vi "getSeries_from_node.vi"(8 "Error IN":errorcluster, 10 "Selected item":string, 11 "HEKAdat.lvclass IN":refnum<class "HEKAdat.lvclass">) -> (0 "Error OUT":errorcluster, 1 "File Parameters OUT":T1, 2 "Traces":sgl[][](array[numeric]), 3 "HEKAdat.lvclass OUT":refnum<class "HEKAdat.lvclass">)   [LabVIEW 2017, in "HEKAdat.lvclass"]
uses:
  HEKAdat.lvclass
  File Parameters.ctl
  HEKAdat.lvclass/HEKAdat.ctl
panel:
  in  "File Parameters":T1
  out "Dim_trace":i32[](array[numeric])
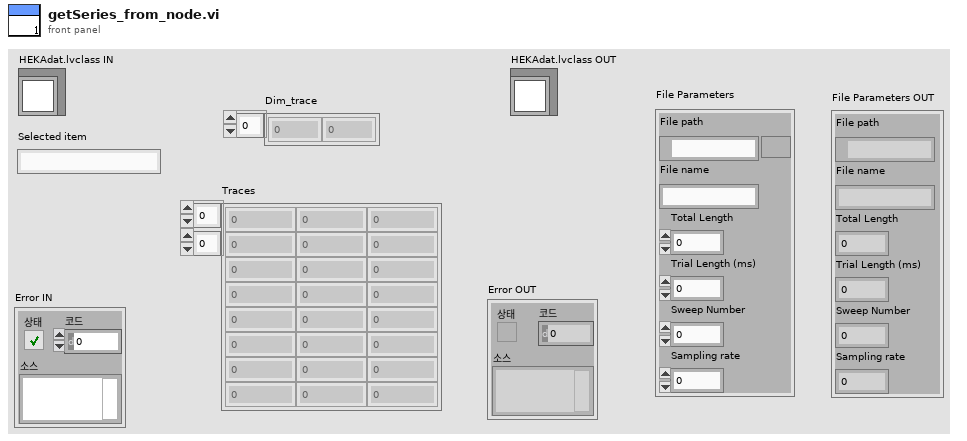
[diagram p1: front panel]
types:
  T1 = typedef "File Parameters.ctl" = cluster{"File path":path, "File name":string, "Total Length":i32, "Trial Length (ms)":dbl, "Sweep Number":dbl, "Sampling rate":dbl}
  T2 = cluster{"Label (Group)":string, "dataptr (Group)":u32, "nchildren (Group)":u32, "Series (1D)":cluster{"Label (Series)":string, "dataptr (Series)":u32, "nchildren (Series)":u32, "Sweep (1D)":cluster{"Label (Sweep)":string, "dataptr (Sweep)":u32, "nchildren (Sweep)":u32, "Trace (1D)":cluster{"dataptr (trace)":u32, "Label (Trace)":string, "Unit":string, "Unit_":dbl, "Xinterval":dbl, "nDatapoints":u32, "offset":u32, "Datascaler":dbl, "Trace":dbl[]}[]}[]}[]}[]
  T3 = cluster{"Label (Group)":string, "dataptr (Group)":u32, "nchildren (Group)":u32, "Series (1D)":cluster{"Label (Series)":string, "dataptr (Series)":u32, "nchildren (Series)":u32, "Sweep (1D)":cluster{"Label (Sweep)":string, "dataptr (Sweep)":u32, "nchildren (Sweep)":u32, "Trace (1D)":cluster{"dataptr (trace)":u32, "Label (Trace)":string, "Unit":string, "Unit_":dbl, "Xinterval":dbl, "nDatapoints":u32, "offset":u32, "Datascaler":dbl, "Trace":dbl[]}[]}[]}[]}
  T4 = cluster{"Label (Series)":string, "dataptr (Series)":u32, "nchildren (Series)":u32, "Sweep (1D)":cluster{"Label (Sweep)":string, "dataptr (Sweep)":u32, "nchildren (Sweep)":u32, "Trace (1D)":cluster{"dataptr (trace)":u32, "Label (Trace)":string, "Unit":string, "Unit_":dbl, "Xinterval":dbl, "nDatapoints":u32, "offset":u32, "Datascaler":dbl, "Trace":dbl[]}[]}[]}[]
  T5 = cluster{"Label (Series)":string, "dataptr (Series)":u32, "nchildren (Series)":u32, "Sweep (1D)":cluster{"Label (Sweep)":string, "dataptr (Sweep)":u32, "nchildren (Sweep)":u32, "Trace (1D)":cluster{"dataptr (trace)":u32, "Label (Trace)":string, "Unit":string, "Unit_":dbl, "Xinterval":dbl, "nDatapoints":u32, "offset":u32, "Datascaler":dbl, "Trace":dbl[]}[]}[]}
  T6 = cluster{"Label (Sweep)":string, "dataptr (Sweep)":u32, "nchildren (Sweep)":u32, "Trace (1D)":cluster{"dataptr (trace)":u32, "Label (Trace)":string, "Unit":string, "Unit_":dbl, "Xinterval":dbl, "nDatapoints":u32, "offset":u32, "Datascaler":dbl, "Trace":dbl[]}[]}[]
  T7 = cluster{"dataptr (trace)":u32, "Label (Trace)":string, "Unit":string, "Unit_":dbl, "Xinterval":dbl, "nDatapoints":u32, "offset":u32, "Datascaler":dbl, "Trace":dbl[]}[]
  T8 = cluster{"dataptr (trace)":u32, "Label (Trace)":string, "Unit":string, "Unit_":dbl, "Xinterval":dbl, "nDatapoints":u32, "offset":u32, "Datascaler":dbl, "Trace":i16[]}
  T9 = cluster{"Label (Sweep)":string, "dataptr (Sweep)":u32, "nchildren (Sweep)":u32, "Trace (1D)":cluster{"dataptr (trace)":u32, "Label (Trace)":string, "Unit":string, "Unit_":dbl, "Xinterval":dbl, "nDatapoints":u32, "offset":u32, "Datascaler":dbl, "Trace":dbl[]}[]}
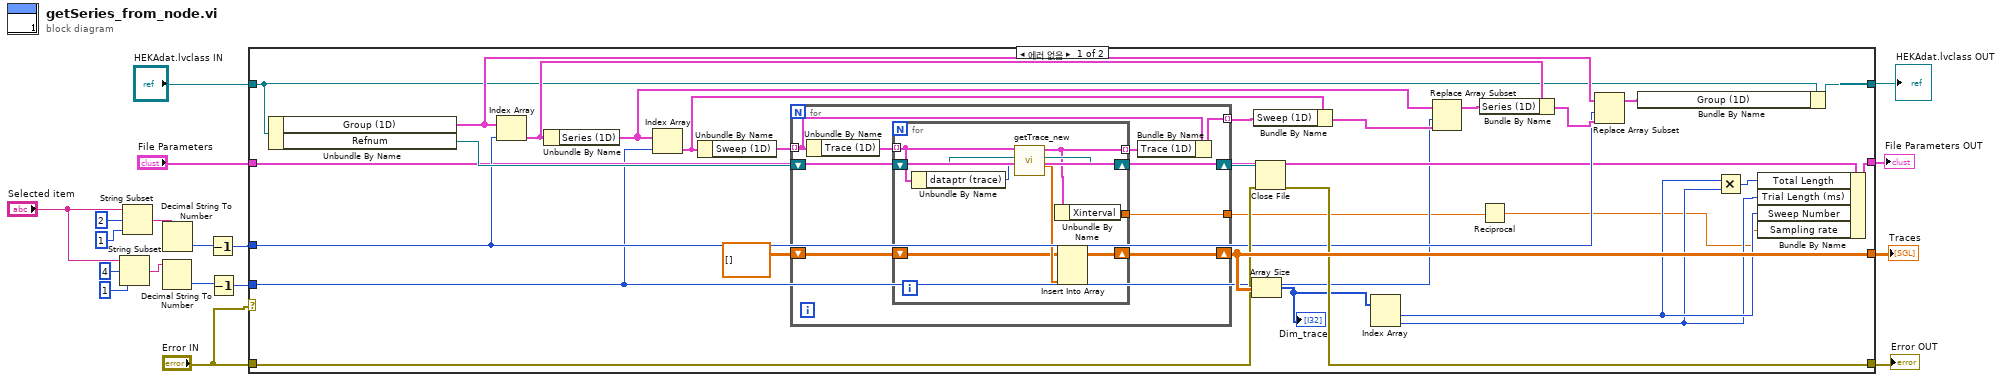
[diagram p0: block diagram]
diagram:
  n1 = String Subset(string="Selected item", offset (0)=4 ("오프셋(0)"), length (rest)=1 ("길이(나머지)")) -> (substring=w7:string)
  n2 = String Subset(string="Selected item", offset (0)=2 ("오프셋(0)"), length (rest)=1 ("길이(나머지)")) -> (substring=w8:string)
  n3 = Decimal String To Number(string=w7) -> (number=w3:i32)  [unwired: 2 in, 1 out]
  n4 = Decimal String To Number(string=w8) -> (number=w6:i32)  [unwired: 2 in, 1 out]
  n5 = Decrement(x=w6) -> (x-1=w5:i32)
  n6 = Decrement(x=w3) -> (x-1=w4:i32)
  n7 = case shown="에러 없음" "Error IN" {
    tunnel: "Error IN" -> [w41 w66]
    tunnel: [w40 w66] -> w17
    tunnel: "HEKAdat.lvclass IN" -> [w29 w65]
    tunnel: [w28 w65] -> w15
    tunnel: w5 -> [w31 _]
    tunnel: w4 -> [w25 _]
    tunnel: [w44 _] -> w14
    tunnel: "File Parameters" -> [w27 _]
    tunnel: [w26 _] -> w1
    frame No Error {
      n8 = Unbundle By Name(w29) -> ("Group (1D)"=w33:T2, "Refnum"=w43:refnum<file>)
      n9 = Index Array(array=w33, index=w31) -> (element=w35:T3)
      n10 = Unbundle By Name(w35) -> ("Series (1D)"=w37:T4)
      n11 = Index Array(array=w37, index=w25) -> (element=w39:T5)
      n12 = Unbundle By Name(w39) -> ("Sweep (1D)"=w46:T6)
      n13 = for {
        tunnel: w46 -> [w50] mode=indexing
        shift-right: [w53] -> w44
        shift-left: sgl[][] [] -> [w52]
        shift-right: [w51] -> w42
        shift-left: w43 -> [w54]
        tunnel: [w48] -> w38 mode=indexing
        tunnel: [w47] -> w20
        n14 = Unbundle By Name(w50) -> ("Trace (1D)"=w55:T7)
        n15 = for {
          tunnel: w55 -> [w59] mode=indexing
          shift-right: [w63] -> w53
          shift-left: w52 -> [w62]
          shift-right: [w61] -> w51
          shift-left: w54 -> [w60]
          tunnel: [w57] -> w49 mode=indexing
          tunnel: [w56] -> w47
          n16 = Unbundle By Name(w59) -> ("dataptr (trace)"=w58:u32)
          n17 = call "getTrace_new.vi"("ptr"=w58, "Refnum IN"=w60, "Trace attribute IN"=w59) -> ("1D array"=w64:sgl[], "refnum OUT"=w61:refnum<file>, "Trace attribute OUT"=w57:T8)  [unwired: 1 in, 1 out]
          n18 = Unbundle By Name(w57) -> ("Xinterval"=w56:dbl)
          n19 = Insert Into Array(array=w62, new element=w64) -> (w63:sgl[][])  [unwired: 2 in]
        }
        n20 = Bundle By Name(cluster=w50, "Trace (1D)"=w49) -> (w48:T9)
      }
      n21 = Array Size(array=w44) -> (size(s)=w24:i32[])
      "Dim_trace" <- w24
      n22 = Bundle By Name(cluster=w39, "Sweep (1D)"=w38) -> (w36:T5)
      n23 = Close File(refnum=w42, error in=w41) -> (error out=w40:errorcluster)  [unwired: 1 out]
      n24 = Index Array(array=w24) -> (element #1=w22:i32, element #2=w21:i32)  [unwired: 2 in]
      n25 = Replace Array Subset(array=w37, new element=w36, index=w25) -> (w34:T4)
      n26 = Bundle By Name(cluster=w35, "Series (1D)"=w34) -> (w32:T3)
      n27 = Reciprocal(x=w20) -> (1/x=w19:dbl)
      n28 = Replace Array Subset(array=w33, new element=w32, index=w31) -> (w30:T2)
      n29 = Bundle By Name(cluster=w29, "Group (1D)"=w30) -> (w28:refnum<class "HEKAdat.lvclass">)
      n30 = Multiply(x=w22, y=w21) -> (x*y=w23:i32)
      n31 = Bundle By Name(cluster=w27, "Total Length"=w23, "Trial Length (ms)"=w21, "Sweep Number"=w22, "Sampling rate"=w19) -> (w26:T1)
    }
    frame Error {
    }
  }
  "Error OUT" <- w17
  "HEKAdat.lvclass OUT" <- w15
  "Traces" <- w14
  "File Parameters OUT" <- w1
